vi "CalibrateOnUserButton.vi"(8 "error in":errorcluster, 11 "Sensors":T1={"Gyro"={"DevStatus"={"status"=FALSE, "code"=0, "source"=""}, "Analog Module"=enum."Controller 1", "Analog Channel"=enum."AI 0", "Offset"=0.0, "Gain (VoltsPerDegree/Second)"=0.0}, "Encoders"={"Left Drive CAN"={"DeviceStatus"={"status"=FALSE, "code"=0, "source"=""}, "Type"=enum."PWM", "PWM"={"Controller"=enum."Controller 1", "PWM Channel"=enum."PWM 0", "DeadBand"={"Name"="", "maxPositivePwm"=0, "minPositivePwm"=0, "centerPwm"=0, "maxNegativePwm"=0, "minNegativePwm"=0, "angularRange"=0}}, "CAN"={"Device Number"=0, "Control Mode"=enum."Percent VBus", "Semaphore"=refnum, "Max Vout"=0.0, "TalonSRX Control Mode"=enum."Percent VBus"}, "Invert"=FALSE, "TransformRef"=refnum, "InvTransformRef"=refnum}, "Right Drive CAN"={"DeviceStatus"={"status"=FALSE, "code"=0, "source"=""}, "Type"=enum."PWM", "PWM"={"Controller"=enum."Controller 1", "PWM Channel"=enum."PWM 0", "DeadBand"={"Name"="", "maxPositivePwm"=0, "minPositivePwm"=0, "centerPwm"=0, "maxNegativePwm"=0, "minNegativePwm"=0, "angularRange"=0}}, "CAN"={"Device Number"=0, "Control Mode"=enum."Percent VBus", "Semaphore"=refnum, "Max Vout"=0.0, "TalonSRX Control Mode"=enum."Percent VBus"}, "Invert"=FALSE, "TransformRef"=refnum, "InvTransformRef"=refnum}, "Strafe CAN"={"DeviceStatus"={"status"=FALSE, "code"=0, "source"=""}, "Type"=enum."PWM", "PWM"={"Controller"=enum."Controller 1", "PWM Channel"=enum."PWM 0", "DeadBand"={"Name"="", "maxPositivePwm"=0, "minPositivePwm"=0, "centerPwm"=0, "maxNegativePwm"=0, "minNegativePwm"=0, "angularRange"=0}}, "CAN"={"Device Number"=0, "Control Mode"=enum."Percent VBus", "Semaphore"=refnum, "Max Vout"=0.0, "TalonSRX Control Mode"=enum."Percent VBus"}, "Invert"=FALSE, "TransformRef"=refnum, "InvTransformRef"=refnum}, "Elevator CAN"={"DeviceStatus"={"status"=FALSE, "code"=0, "source"=""}, "Type"=enum."PWM", "PWM"={"Controller"=enum."Controller 1", "PWM Channel"=enum."PWM 0", "DeadBand"={"Name"="", "maxPositivePwm"=0, "minPositivePwm"=0, "centerPwm"=0, "maxNegativePwm"=0, "minNegativePwm"=0, "angularRange"=0}}, "CAN"={"Device Number"=0, "Control Mode"=enum."Percent VBus", "Semaphore"=refnum, "Max Vout"=0.0, "TalonSRX Control Mode"=enum."Percent VBus"}, "Invert"=FALSE, "TransformRef"=refnum, "InvTransformRef"=refnum}}, "Switches"={"Elevator Top"={"DevStatus"={"status"=FALSE, "code"=0, "source"=""}, "DIO Channel"=enum."DIO 0", "Controller"=enum."Controller 1", "CntIndex"=enum."Ctr 0", "Normally Closed"=FALSE}, "Elevator Bottom"={"DevStatus"={"status"=FALSE, "code"=0, "source"=""}, "DIO Channel"=enum."DIO 0", "Controller"=enum."Controller 1", "CntIndex"=enum."Ctr 0", "Normally Closed"=FALSE}, "Claw Outside"={"DevStatus"={"status"=FALSE, "code"=0, "source"=""}, "DIO Channel"=enum."DIO 0", "Controller"=enum."Controller 1", "CntIndex"=enum."Ctr 0", "Normally Closed"=FALSE}, "Tote Touch"={"DevStatus"={"status"=FALSE, "code"=0, "source"=""}, "DIO Channel"=enum."DIO 1", "Controller"=enum."Controller 1", "CntIndex"=enum."Invalid", "Normally Closed"=FALSE}}, "Arm Capper Pot"={"DevStatus"={"status"=FALSE, "code"=0, "source"=""}, "Controller"=enum."Controller 1", "Analog Channel"=enum."AI 0", "Invert Output"=FALSE}, "Arm Angle Pot"={"DevStatus"={"status"=FALSE, "code"=0, "source"=""}, "Controller"=enum."Controller 1", "Analog Channel"=enum."AI 0", "Invert Output"=FALSE}, "Sonar"={"Front"={"AIDeviceRef"={"DevStatus"={"status"=FALSE, "code"=0, "source"=""}, "Controller"=enum."Controller 1", "Analog Channel"=enum."Invalid"}, "Scaling factor (V/in)"=0.0098, "Average Bits"=3}, "Back"={"AIDeviceRef"={"DevStatus"={"status"=FALSE, "code"=0, "source"=""}, "Controller"=enum."Controller 1", "Analog Channel"=enum."Invalid"}, "Scaling factor (V/in)"=0.0098, "Average Bits"=3}}} {"Sonar"."Back"."Average Bits" max=15; "Sonar"."Front"."Average Bits" max=15}) -> ()   [LabVIEW 2014]
uses:
  Utilities/Sensors.ctl
  <vilib>/Rock Robotics/WPI/Gyro/WPI_GyroDevRef.ctl
  <vilib>/Rock Robotics/SystemInterfaces/Typedef/FPGA_TypedefAnalogModule.ctl
  <vilib>/Rock Robotics/SystemInterfaces/AI/FPGA_AIChannel.ctl
  <vilib>/Rock Robotics/WPI/MotorControl/WPI_MotorControlDeviceRef.ctl
  <vilib>/Rock Robotics/WPI/MotorControl/WPI_MotorControlType.ctl
  <vilib>/Rock Robotics/SystemInterfaces/Typedef/FPGA_TypedefDigitalModule.ctl
  <vilib>/Rock Robotics/SystemInterfaces/DIO/FPGA_DIOPWMChannel.ctl
  <vilib>/Rock Robotics/WPI/PWM/WPI_PWMDeadband.ctl
  <vilib>/Rock Robotics/WPI/CAN/Jaguar/SubVIs/WPI_CANJaguar_ControlMode.ctl
  <vilib>/Rock Robotics/WPI/CAN/TalonSRX/WPI_CANTalonSRX_APIControlMode.ctl
  <vilib>/Rock Robotics/WPI/PWM/WPI_PWMTransform_ConPane.ctl
  <vilib>/Rock Robotics/WPI/Switch/WPI_SwitchDevRef.ctl
  <vilib>/Rock Robotics/SystemInterfaces/DIO/FPGA_DIOChannel.ctl
  <vilib>/Rock Robotics/SystemInterfaces/Counter/FPGA_CounterCtrSystemIndex.ctl
  <vilib>/Rock Robotics/WPI/Potentiometer/WPI_PotentiometerDevRef.ctl
  <vilib>/Rock Robotics/WPI/Ultrasonic/WPI_SonarMB1010AnalogDeviceRef.ctl
  <vilib>/Rock Robotics/WPI/AnalogChannel/WPI_AnalogChannelDevRef.ctl
  <vilib>/Rock Robotics/SystemInterfaces/Typedef/FPGA_TypedefAnalogModuleForGyro.ctl
  <vilib>/Rock Robotics/SystemInterfaces/AI/FPGA_AIGyroChannel.ctl
  <vilib>/Rock Robotics/SystemInterfaces/AI/FPGA_AIDevRef.ctl
panel:
  out "Angle 2":dbl(knob) scale=0.0..360.0
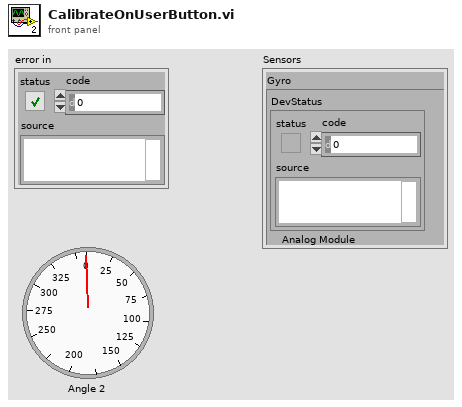
[diagram p1: front panel]
types:
  T1 = typedef "Sensors.ctl" = cluster{"Gyro":T2, "Encoders":cluster{"Left Drive CAN":T5, "Right Drive CAN":T5, "Strafe CAN":T5, "Elevator CAN":T5}, "Switches":cluster{"Elevator Top":T14, "Elevator Bottom":T14, "Claw Outside":T14, "Tote Touch":T14}, "Arm Capper Pot":T17, "Arm Angle Pot":T17, "Sonar":cluster{"Front":T18, "Back":T18}}
  T2 = typedef "WPI_GyroDevRef.ctl" = cluster{"DevStatus":errorcluster, "Analog Module":T3, "Analog Channel":T4, "Offset":dbl, "Gain (VoltsPerDegree/Second)":dbl}
  T3 = typedef "FPGA_TypedefAnalogModule.ctl" = enum16{"Controller 1"}
  T4 = typedef "FPGA_AIChannel.ctl" = enum8{"AI 0", "AI 1", "AI 2", "AI 3", "AI MXP 0", "AI MXP 1", "AI MXP 2", "AI MXP 3", "Invalid"}
  T5 = typedef "WPI_MotorControlDeviceRef.ctl" = cluster{"DeviceStatus":errorcluster, "Type":T6, "PWM":cluster{"Controller":T7, "PWM Channel":T8, "DeadBand":T9}, "CAN":cluster{"Device Number":u8, "Control Mode":T10, "Semaphore":T11, "Max Vout":dbl, "TalonSRX Control Mode":T12}, "Invert":bool, "TransformRef":T13, "InvTransformRef":T13}
  T6 = typedef "WPI_MotorControlType.ctl" = enum16{"PWM", "CAN", "CANTalonSRX"}
  T7 = typedef "FPGA_TypedefDigitalModule.ctl" = enum16{"Controller 1"}
  T8 = typedef "FPGA_DIOPWMChannel.ctl" = enum8{"PWM 0", "PWM 1", "PWM 2", "PWM 3", "PWM 4", "PWM 5", "PWM 6", "PWM 7", "PWM 8", "PWM 9", "PWM MXP 0", "PWM MXP 1", "PWM MXP 2", "PWM MXP 3", "PWM MXP 4", "PWM MXP 5", "PWM MXP 6", "PWM MXP 7", "PWM MXP 8", "PWM MXP 9", "Invalid"}
  T9 = typedef "WPI_PWMDeadband.ctl" = cluster{"Name":string, "maxPositivePwm":i32, "minPositivePwm":i32, "centerPwm":i32, "maxNegativePwm":i32, "minNegativePwm":i32, "angularRange":u16}
  T10 = typedef "WPI_CANJaguar_ControlMode.ctl" = enum8{"Percent VBus", "Current", "Speed", "Position", "Voltage"}
  T11 = typedef "Semaphore RefNum" = refnum<k1>
  T12 = typedef "WPI_CANTalonSRX_APIControlMode.ctl" = enum8{"Percent VBus", "Speed", "Position", "Slave", "Unchanged / Invalid"}
  T13 = typedef "WPI_PWMTransform_ConPane.ctl" = refnum<vi>
  T14 = typedef "WPI_SwitchDevRef.ctl" = cluster{"DevStatus":errorcluster, "DIO Channel":T15, "Controller":T7, "CntIndex":T16, "Normally Closed":bool}
  T15 = typedef "FPGA_DIOChannel.ctl" = enum8{"DIO 0", "DIO 1", "DIO 2", "DIO 3", "DIO 4", "DIO 5", "DIO 6", "DIO 7", "DIO 8", "DIO 9", "DIO MXP 0", "DIO MXP 1", "DIO MXP 2", "DIO MXP 3", "DIO MXP 4", "DIO MXP 5", "DIO MXP 6", "DIO MXP 7", "DIO MXP 8", "DIO MXP 9", "DIO MXP 10", "DIO MXP 11", "DIO MXP 12", "DIO MXP 13", "DIO MXP 14", "DIO MXP 15", "Invalid"}
  T16 = typedef "FPGA_CounterCtrSystemIndex.ctl" = enum8{"Ctr 0", "Ctr 1", "Ctr 2", "Ctr 3", "Ctr 4", "Ctr 5", "Ctr 6", "Ctr 7", "Invalid"}
  T17 = typedef "WPI_PotentiometerDevRef.ctl" = cluster{"DevStatus":errorcluster, "Controller":T3, "Analog Channel":T4, "Invert Output":bool}
  T18 = typedef "WPI_SonarMB1010AnalogDeviceRef.ctl" = cluster{"AIDeviceRef":T19, "Scaling factor (V/in)":dbl, "Average Bits":u8}
  T19 = typedef "WPI_AnalogChannelDevRef.ctl" = cluster{"DevStatus":errorcluster, "Controller":T3, "Analog Channel":T4}
  T20 = typedef "FPGA_AIGyroChannel.ctl" = enum8{"AI 0", "AI 1", "Invalid"}
  T21 = typedef "FPGA_TypedefAnalogModuleForGyro.ctl" = enum16{"Controller 1"}
  T22 = typedef "FPGA_AIDevRef.ctl" = cluster{"DevStatus":errorcluster, "Controller":T3}
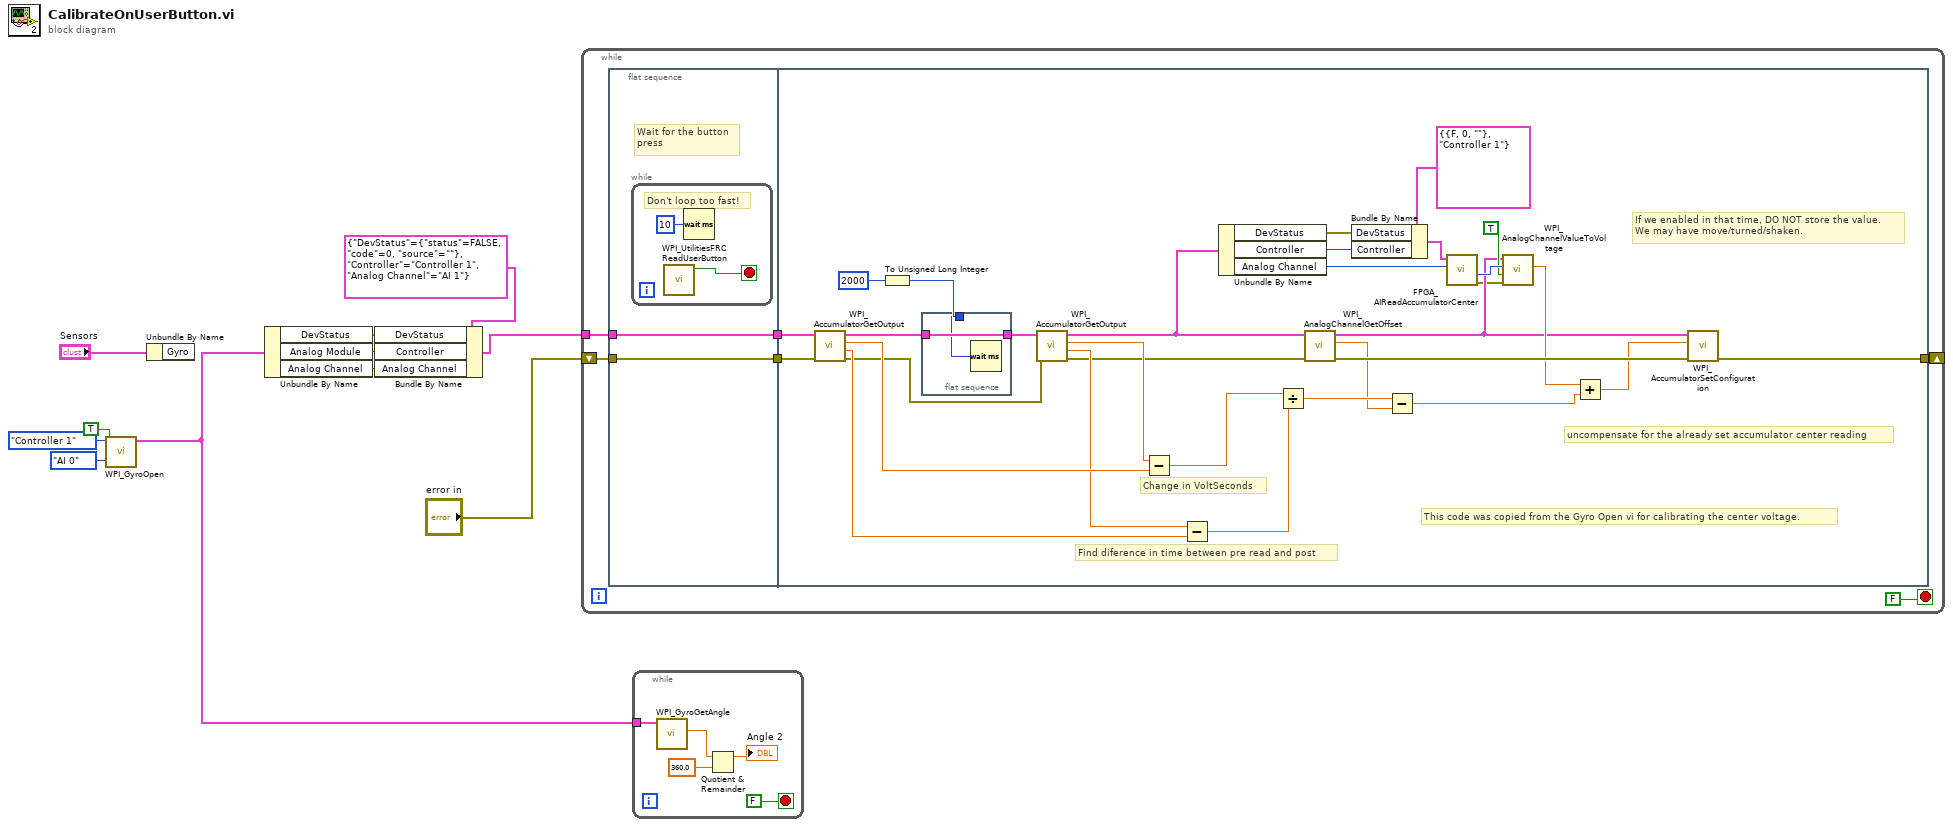
[diagram p0: block diagram]
diagram:
  n1 = call <vilib>:"WPI_GyroOpen.vi"("Calibrate On Open"=TRUE, "Analog Channel"=FPGA_AIGyroChannel."AI 0", "Controller"=FPGA_TypedefAnalogModuleForGyro."Controller 1") -> ("GyroDevRef"=w4:T2)  [unwired: 6 in, 2 out]
  n2 = Unbundle By Name("Sensors") -> ()  [unwired: 1 out]
  n3 = Unbundle By Name(w4) -> ("DevStatus"=w10:errorcluster, "Analog Module"=w9:T3, "Analog Channel"=w8:T4)
  n4 = Bundle By Name(cluster=T19 {"DevStatus"={"status"=FALSE, "code"=0, "source"=""}, "Controller"=enum."Controller 1", "Analog Channel"=enum."AI 1"} ("AIDeviceRef"), "DevStatus"=w10, "Controller"=w9, "Analog Channel"=w8) -> (w6:T19)
  n5 = while {
    tunnel: w6 -> [w17]
    shift-right: [w15] -> _
    shift-left: "error in" -> [w16]
    stop <- FALSE stop-if-true
    n6 = flat-sequence {
      tunnel: w16 -> [w18]
      tunnel: w17 -> [w19]
      tunnel: [w19] -> w13
      tunnel: [w18] -> w12
      tunnel: [w22] -> w15
      tunnel: w13 -> [w24]
      tunnel: w12 -> [w23]
      frame #0 {
        # "Wait for the button\npress"
        n7 = while {
          stop <- w21 stop-if-true
          # "Don't loop too fast!"
          n8 = call <vilib>:"WPI_UtilitiesFRC ReadUserButton.vi"() -> ("User Button"=w21:bool)  [unwired: 10 in, 1 out]
          n9 = Wait (ms)(milliseconds to wait=u32 10) -> ()  [unwired: 1 out]
        }
      }
      frame #1 {
        # "uncompensate for the already set accumulator center reading"
        # "Change in VoltSeconds"
        # "Find diference in time between pre read and post"
        # "This code was copied from the Gyro Open vi for calibrating the center voltage."
        # "If we enabled in that time, DO NOT store the value.\nWe may have move/turned/shaken."
        n10 = call <vilib>:"WPI_AccumulatorGetOutput.vi"("error in (no error)"=w23, "AIDeviceRef"=w24) -> ("error out"=w40:errorcluster, "Duration (Seconds)"=w49:dbl, "Value (Volt Seconds)"=w48:dbl, "AIDeviceRef"=w50:T19)  [unwired: 6 out]
        n11 = To Unsigned Long Integer(number=u32 2000) -> (unsigned 32bit integer=w51:u32)
        n12 = flat-sequence {
          tunnel: w50 -> [w54]
          tunnel: w51 -> [w53]
          tunnel: [w54] -> w39
          frame #0 {
            n13 = Wait (ms)(milliseconds to wait=w53) -> ()  [unwired: 1 out]
          }
        }
        n14 = call <vilib>:"WPI_AccumulatorGetOutput.vi"("error in (no error)"=w40, "AIDeviceRef"=w39) -> ("error out"=w41:errorcluster, "Duration (Seconds)"=w45:dbl, "Value (Volt Seconds)"=w47:dbl, "AIDeviceRef"=w34:T19)  [unwired: 6 out]
        n15 = Subtract(x=w47, y=w48) -> (x-y=w46:dbl)
        n16 = Subtract(x=w45, y=w49) -> (x-y=w44:dbl)
        n17 = Unbundle By Name(w34) -> ("DevStatus"=w30:errorcluster, "Controller"=w29:T3, "Analog Channel"=w33:T4)
        n18 = Divide(x=w46, y=w44) -> (x/y=w52:dbl)
        n19 = call <vilib>:"WPI_AnalogChannelGetOffset.vi"("error in (no error)"=w41, "AIDeviceRef"=w34) -> ("error out"=w43:errorcluster, "Offset"=w42:dbl, "AIDeviceRef"=w35:T19)  [unwired: 7 out]
        n20 = Bundle By Name(cluster=T22 {"DevStatus"={"status"=FALSE, "code"=0, "source"=""}, "Controller"=enum."Controller 1"} ("AI Reference in"), "DevStatus"=w30, "Controller"=w29) -> (w28:T22)
        n21 = Subtract(x=w52, y=w42) -> (x-y=w27:dbl)
        n22 = call <vilib>:"FPGA_AIReadAccumulatorCenter.vi"("Channel"=w33, "AI Reference in"=w28) -> ("error out"=w32:errorcluster, "Center"=w38:i32)  [unwired: 7 in, 1 out]
        n23 = call <vilib>:"WPI_AnalogChannelValueToVoltage.vi"("error in (no error)"=w32, "Averaged"=TRUE, "Value"=w38, "AIDeviceRef"=w35) -> ("Voltage"=w37:dbl)  [unwired: 5 in, 2 out]
        n24 = Add(x=w37, y=w27) -> (x+y=w26:dbl)
        n25 = call <vilib>:"WPI_AccumulatorSetConfiguration.vi"("error in (no error)"=w43, "Center"=w26, "AIDeviceRef"=w35) -> ("error out"=w22:errorcluster)  [unwired: 2 in, 6 out]
      }
    }
  }
  n26 = while {
    tunnel: w4 -> [w59]
    stop <- FALSE stop-if-true
    n27 = call <vilib>:"WPI_GyroGetAngle.vi"("GyroDevRef"=w59) -> ("Angle"=w56:dbl)  [unwired: 7 in, 3 out]
    n28 = Quotient & Remainder(x=w56, y=360.0) -> (x-y*floor(x/y)=→"Angle 2":dbl)  [unwired: 1 out]
  }
